vi "UDP Receiver.vi"() -> ()   [LabVIEW 2012]
panel:
  in  "reset":bool
  in  "stop":bool
  out "Data Received":string
  in  "max bytes/read":i32=548
  out "# of Bytes Received":i32
  in  "Port":u16=58432
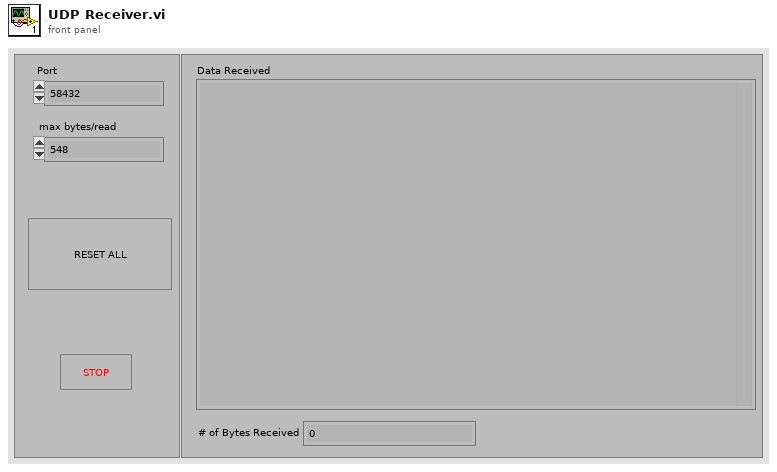
[diagram p1: front panel]
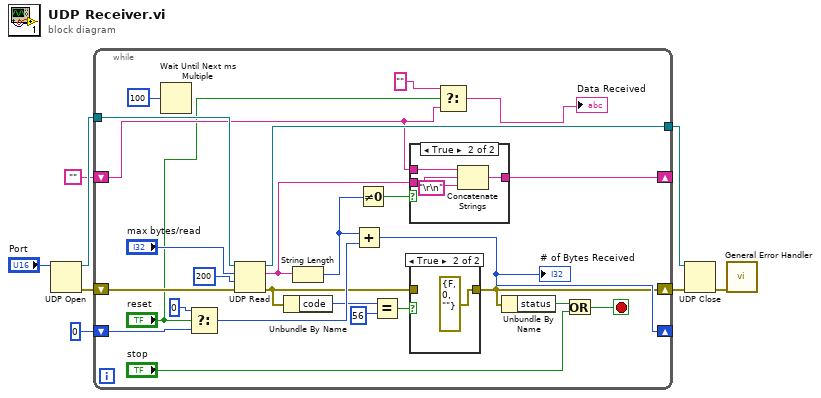
[diagram p0: block diagram]
diagram:
  n1 = UDP Open(11:"Port") -> (port=w6:refnum<k16>, 0:w7:errorcluster)  [unwired: 4 in, 1 out]
  n2 = while {
    shift-left: "" -> [w12]
    shift-right: [w20] -> _
    shift-left: 0 -> [w25]
    shift-right: [w26] -> _
    tunnel: [w32] -> w5
    tunnel: w6 -> [w33]
    shift-left: w7 -> [w34]
    shift-right: [w14] -> w4
    stop <- w29 stop-if-true
    n3 = Wait Until Next ms Multiple(millisecond multiple=u32 100) -> ()  [unwired: 1 out]
    n4 = Select(t=0, s="reset", f=w25) -> (s? t:f=w24:i32)
    n5 = UDP Read(connection ID=w33, max size (548)="max bytes/read", timeout ms (25000)=200, 8:w34) -> (data out=w21:string, error out=w13:errorcluster, 3:w32:refnum<k16>)  [unwired: 2 out]
    n6 = Unbundle By Name(w13) -> ("code"=w17:i32)
    n7 = String Length(string=w21) -> (length=w19:i32)
    n8 = Add(x=w19, y=w24) -> (x+y=w26:i32)
    "# of Bytes Received" <- w26
    n9 = Not Equal To 0?(x=w19) -> (x != 0?=w18:bool)
    n10 = Equal?(x=w17, y=56) -> (x = y?=w15:bool)
    n11 = case shown="True" w18 {
      tunnel: w12 -> [w37 w41]
      tunnel: w21 -> [_ w39]
      tunnel: [w37 w40] -> w20
      frame False {
      }
      frame True {
        n12 = Concatenate Strings(w41, w39, "\r\n" ("Substring")) -> (w40:string)
      }
    }
    n13 = case shown="True" w15 {
      tunnel: w13 -> [w35 _]
      tunnel: [w35 errorcluster {"status"=FALSE, "code"=0, "source"=""} ("error out")] -> w14
      frame False {
      }
      frame True {
      }
    }
    n14 = Select(t="" ("source"), s="reset", f=w12) -> (s? t:f=→"Data Received":string)
    n15 = Unbundle By Name(w14) -> ("status"=w28:bool)
    n16 = Or(x=w28, y="stop") -> (x .or. y?=w29:bool)
  }
  n17 = UDP Close(connection ID=w5, 8:w4) -> (error out=w3:errorcluster)  [unwired: 1 out]
  n18 = call <vilib>:"General Error Handler.vi"("error in (no error)"=w3) -> ()  [unwired: 10 in, 5 out]
